vi "Handle Errors.vi"(8 "error in":errorcluster, 11 "Instrument in":refnum<class "Instrument.lvclass">) -> (0 "error out":errorcluster, 2 "errors":errorcluster[](array[cluster]), 3 "Instrument out":refnum<class "Instrument.lvclass">)   [LabVIEW 2014, in "Instrument.lvclass"]
doc: "Dequeue errors here and make them available through the <B>errors</B> node. The <B>Error to Handle?</B> flag will be cleared to prevent this VI from being called erroneously."
uses:
  Instrument.lvclass
  Instrument.lvclass/Instrument.ctl
  Session APIs/Session Log/System Log.lvclass
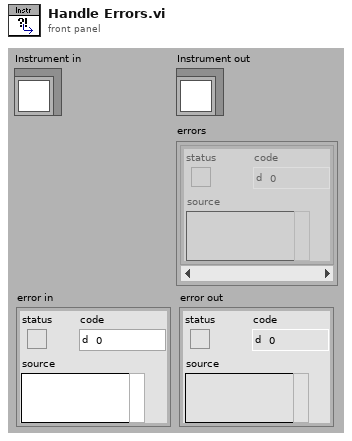
[diagram p1: front panel]
types:
  T1 = typedef "Session - Root.lvclass/Session Handle.ctl" = refnum<data-value>
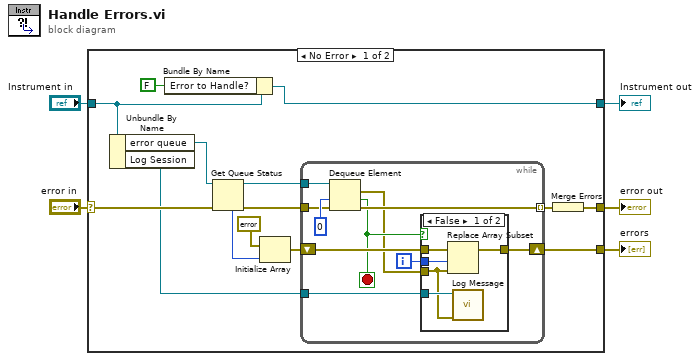
[diagram p0: block diagram]
diagram:
  n1 = case shown="No Error" "error in" {
    selector: "error in" -> [w15 w37]
    tunnel: [w18 w37] -> w4
    tunnel: [w7 w36] -> w2
    tunnel: "Instrument in" -> [w9 w36]
    tunnel: [w10 _] -> w1
    frame No Error {
      n2 = Unbundle By Name(w9) -> ("error queue"=w17:refnum<queue>, "Log Session"=w6:T1)
      n3 = Bundle By Name(cluster=w9, "Error to Handle?"=FALSE) -> (w7:refnum<class "Instrument.lvclass">)
      n4 = Get Queue Status(queue=w17, error in (no error)=w15) -> (queue out=w16:refnum<queue>, error out=w14:errorcluster, # elements in queue=w13:i32)  [unwired: 1 in, 5 out]
      n5 = Initialize Array(errorcluster {"status"=FALSE, "code"=0, "source"=""} ("error out"), w13) -> (w11:errorcluster[])
      n6 = while {
        tunnel: w16 -> [w29]
        tunnel: w14 -> [w27]
        tunnel: [w26] -> w19 mode=indexing
        shift-right: [w23] -> w10
        shift-left: w11 -> [w25]
        tunnel: w6 -> [w20]
        i -> [w24]
        stop <- w22 stop-if-true
        n7 = Dequeue Element(queue=w29, timeout in ms (-1)=0, error in (no error)=w27) -> (element=w21:errorcluster, timed out?=w22:bool, error out=w26:errorcluster)  [unwired: 1 out]
        n8 = case shown="False" w22 {
          tunnel: w25 -> [w34 w35]
          tunnel: w24 -> [w33 _]
          tunnel: w21 -> [w30 _]
          tunnel: [w32 w35] -> w23
          tunnel: w20 -> [w31 _]
          frame False {
            n9 = Replace Array Subset(array=w34, new element=w30, index=w33) -> (w32:errorcluster[])
            n10 = call "Log Message.vi"("error in"=w30, "session in"=w31) -> ()  [unwired: 8 in, 2 out]
          }
          frame True {
          }
        }
      }
      n11 = Merge Errors(w19) -> (w18:errorcluster)
    }
    frame Error {
    }
  }
  "error out" <- w4
  "Instrument out" <- w2
  "errors" <- w1
